vi "Read Hardware.vi"(8 "error in":errorcluster, 11 "Sensor & Control in":refnum<class "Sensor & Control.lvclass">) -> (0 "error out":errorcluster, 3 "Sensor & Control out":refnum<class "Sensor & Control.lvclass">)   [LabVIEW 2013, in "Sensor & Control.lvlib" / "Sensor & Control.lvclass"]
uses:
  Sensor & Control.lvclass
  Sensor & Control.lvclass/Sensor & Control.ctl
  Read VISA.vi
  Read Value.vi
  PluginInterface/PluginInterface.lvlibp/PluginInterfaceClass/Read Name.vi
  PluginInterface/PluginInterface.lvlibp/PluginInterfaceClass/Read DVR.vi
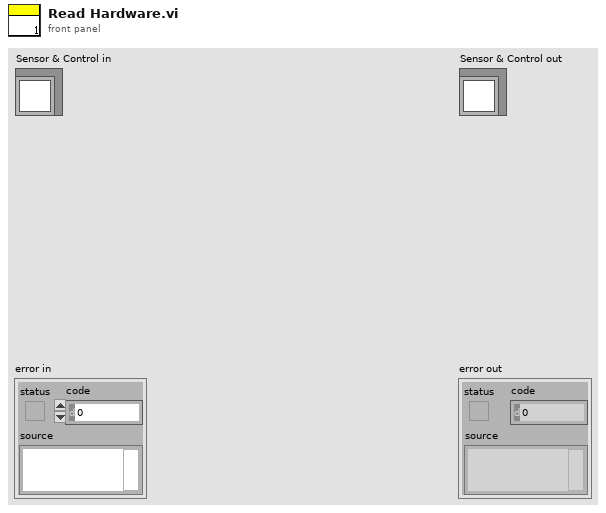
[diagram p1: front panel]
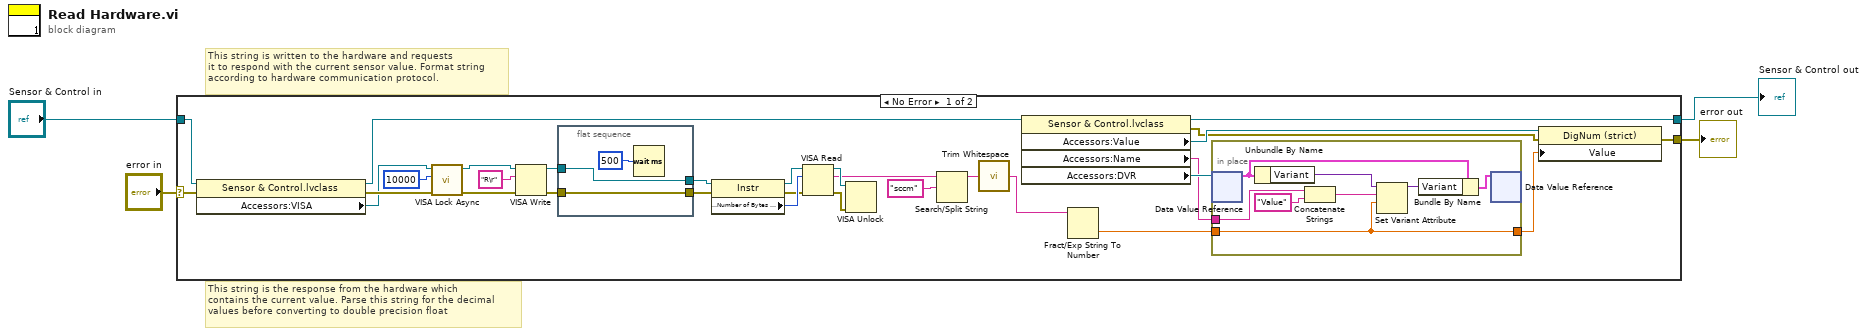
[diagram p0: block diagram]
diagram:
  # "This string is the response from the hardware which\ncontains the current value. Parse this string for the decimal \nvalues before converting to double precision float"
  # "This string is written to the hardware and requests\nit to respond with the current sensor value. Format string\naccording to hardware communication protocol."
  n1 = case shown="No Error" "error in" {
    selector: "error in" -> [w33 w47]
    tunnel: [w25 w47] -> w3
    tunnel: [w5 w46] -> w1
    tunnel: "Sensor & Control in" -> [w34 w46]
    frame No Error {
      n2 = property class="Sensor & Control.lvclass"(reference=w34, error in=w33) -> (reference out=w27:refnum<class "Sensor & Control.lvclass">, error out=w29:errorcluster, "Accessors:VISA"=w28:refnum<visa-resource-name>)
      n3 = call <vilib>:"VISA Lock Async.vi"("error in (no error)"=w29, "timeout (0)"=u32 10000, "VISA resource name"=w28) -> ("error out"=w15:errorcluster, "VISA resource name out"=w16:refnum<visa-resource-name>)  [unwired: 6 in, 1 out]
      n4 = VISA Write(VISA resource name=w16, write buffer="R\r", error in (no error)=w15) -> (VISA resource name out=w24:refnum<visa-resource-name>, error out=w23:errorcluster)  [unwired: 1 out]
      n5 = flat-sequence {
        tunnel: w24 -> [w37]
        tunnel: [w37] -> w18
        tunnel: [w36] -> w22
        tunnel: w23 -> [w36]
        frame #0 {
          n6 = Wait (ms)(milliseconds to wait=u32 500 ("ms before read")) -> ()  [unwired: 1 out]
        }
      }
      n7 = property class="Instr"(reference=w18, error in=w22) -> (reference out=w21:refnum<visa-resource-name>, error out=w19:errorcluster, "Serial Settings:Number of Bytes at Serial Port"=w20:u32)
      n8 = VISA Read(VISA resource name=w21, byte count=w20, error in (no error)=w19) -> (VISA resource name out=w10:refnum<visa-resource-name>, read buffer=w9:string, error out=w11:errorcluster)  [unwired: 1 out]
      n9 = VISA Unlock(8:w11, 11:w10) -> ()  [unwired: 2 out]
      n10 = Search/Split String(string=w9, search string/char (-)="sccm") -> (substring before match=w13:string)  [unwired: 1 in, 2 out]
      n11 = call <vilib>:"Trim Whitespace.vi"("string"=w13) -> ("trimmed string"=w8:string)  [unwired: 1 in]
      n12 = property class="Sensor & Control.lvclass"(reference=w27) -> (reference out=w5:refnum<class "Sensor & Control.lvclass">, error out=w6:errorcluster, "Accessors:Value"=w31:refnum<vi>, "Accessors:Name"=w7:string, "Accessors:DVR"=w32:refnum<data-value>)  [unwired: 1 in]
      n13 = Fract/Exp String To Number(string=w8) -> (number=w26:dbl)  [unwired: 3 in, 1 out]
      n14 = in-place {
        in-place-border: w26 -> [w41]
        in-place-border: [w41] -> w30
        in-place-border: w7 -> [w39]
        n15 = in-place-dvr #1(w32) -> (w42:cluster{"Array":string[], "Variant":variant})  [unwired: 1 out]
        n16 = Unbundle By Name(w42) -> ("Variant"=w44:variant)
        n17 = Concatenate Strings(w39, "Value") -> (w38:string)
        n18 = Set Variant Attribute(Variant=w44, name=w38, value=w41) -> (Variant out=w43:variant)  [unwired: 1 in, 2 out]
        n19 = Bundle By Name(cluster=w42, "Variant"=w43) -> (w45:cluster{"Array":string[], "Variant":variant})
        n20 = in-place-dvr #1(w45) -> ()  [unwired: 2 out]
      }
      n21 = property class="DigNum (strict)"(reference=w31, error in=w6, "Value"=w30) -> (error out=w25:errorcluster)  [unwired: 1 out]
    }
    frame Error {
    }
  }
  "error out" <- w3
  "Sensor & Control out" <- w1
